vi "add.vi"() -> ()   [LabVIEW 2021]
panel:
  out "x+y":dbl
  in  "x":dbl
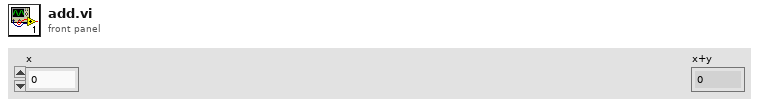
[diagram p1: front panel]
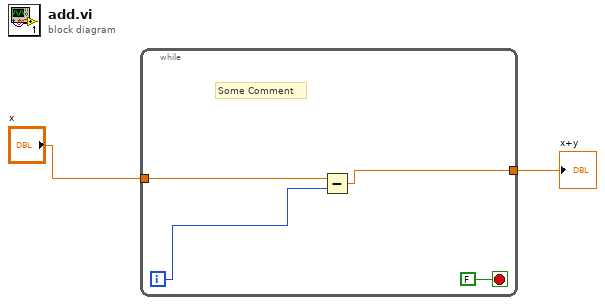
[diagram p0: block diagram]
diagram:
  n1 = while {
    tunnel: "x" -> [w4]
    tunnel: [w3] -> w1
    i -> [w5]
    stop <- FALSE stop-if-true
    # "Some Comment"
    n2 = Subtract(x=w4, y=w5) -> (x-y=w3:dbl)
  }
  "x+y" <- w1
